vi "Init.vi"(8 "error in (no error)":errorcluster, 11 "Tamer in":refnum<class "Tamer.lvclass">) -> (0 "error out":errorcluster, 3 "Tamer out":refnum<class "Tamer.lvclass">)   [LabVIEW 2020, in "Tamer.lvlib" / "Tamer.lvclass"]
uses:
  Tamer.lvclass
  Tamer Consumer Case Selector.ctl
  Classes/Log/Log.lvclass
  Father of all uServices/Father of all uServices/Father of all uServices.lvclass
  TALOS.lvlib
  Ancestor/Ancestor/Infinite Message Selector.ctl
  Ancestor/Ancestor/Ancestor.lvclass
  C:/Users/marco/Documents/GitHub_Lab/TALOS/talos/Father of all uServices/Father of all uServices/Father of all uServices.lvclass
  C:/Users/marco/Documents/GitHub_Lab/TALOS/talos/Ancestor/Ancestor/Ancestor.lvclass
  C:/Users/marco/Documents/GitHub_Lab/TALOS/builds/Actor Framework PPL/Actor Framework.lvlibp/1abvi3w/vi.lib/ActorFramework/Actor/Actor.lvclass
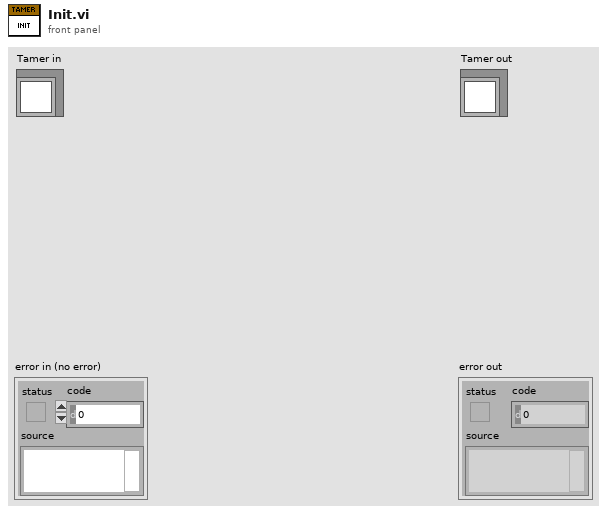
[diagram p1: front panel]
types:
  T1 = typedef "Tamer.lvlib/Tamer.lvclass/Tamer Consumer Case Selector.ctl" = enum16{"New schedule", "Initiate RUN", "Parse Schedules", "Script Checker", "Banana after Quality Check", "Update Crit Lvl", "Propagate Banana", "Reply from Guardian", "Reply from uService", "Timeout of RUN", "uService Replies Check", "Update from Monkey", "Monkey Died", "Reschedule", "Rerun", "Stop DAQ", "Stop Schedule", "Skip Run", "Kill Process", "Update GV"}
  T2 = typedef "TALOS.lvlib/Ancestor.lvlib/Ancestor.lvclass/Infinite Message Selector.ctl" = enum16{"Start", "Stop", "Check", "Flush (Stop all)", "Init"}
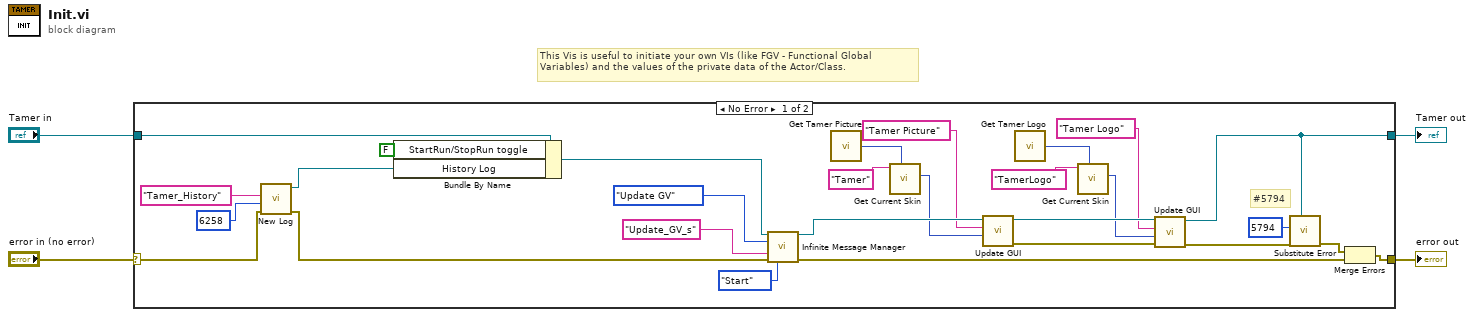
[diagram p0: block diagram]
diagram:
  # "This Vis is useful to initiate your own VIs (like FGV - Functional Global Variables) and the values of the private data of the Actor/Class."
  n1 = case shown="No Error" "error in (no error)" {
    selector: "error in (no error)" -> [w19 w33]
    tunnel: "Tamer in" -> [w24 w34]
    tunnel: [w6 w34] -> w4
    tunnel: [w32 w33] -> w3
    frame No Error {
      # "#5794"
      n2 = call "New Log.vi"("error in (no error)"=w19, "Specific Error Code"=6258, "Name"="Tamer_History") -> ("error out"=w18:errorcluster, "Log out"=w20:refnum<class "Log.lvclass">)  [unwired: 7 in]
      n3 = Bundle By Name(cluster=w24, "StartRun/StopRun toggle"=FALSE ("StartRun already given?"), "History Log"=w20) -> (w25:refnum<class "Tamer.lvclass">)
      n4 = call-dynamic "Infinite Message Manager.vi"("Father of all uServices in"=w25, "Consumer Case Selector"=Tamer_Consumer_Case_Selector."Update GV" ("Monkey Consumer Case Selector"), "Tau parameter"="Update_GV_s", "error in (no error)"=w18, "Infinite Message Selector"=Infinite_Message_Selector."Start") -> ("Father of all uServices out"=w27:refnum<class "Tamer.lvclass">, "error out"=w28:errorcluster)  [unwired: 8 in, 1 out]
      n5 = call "Get Tamer Picture.vi"() -> ("Tamer"=w11:picture)
      n6 = call "Get Current Skin.vi"("default"=w11, "Object"="Tamer") -> ("Picture with skin"=w14:picture)  [unwired: 4 in, 2 out]
      n7 = call "Update GUI.vi"("Data"=w14, "GUI Item Name"="Tamer Picture", "uService Template in"=w27) -> ("error out"=w12:errorcluster, "uService Template out"=w13:refnum<class "Tamer.lvclass">)  [unwired: 7 in]
      n8 = call "Get Tamer Logo.vi"() -> ("Tamer Logo"=w9:picture)
      n9 = call "Get Current Skin.vi"("default"=w9, "Object"="TamerLogo") -> ("Picture with skin"=w8:picture)  [unwired: 4 in, 2 out]
      n10 = call "Update GUI.vi"("error in (no error)"=w12, "Data"=w8, "GUI Item Name"="Tamer Logo", "uService Template in"=w13) -> ("error out"=w5:errorcluster, "uService Template out"=w6:refnum<class "Tamer.lvclass">)  [unwired: 6 in]
      n11 = call "Substitute Error.vi"("LabVIEW Object"=w6, "error in (no error)"=w5, "Error Code"=5794) -> ("error out"=w31:errorcluster)  [unwired: 8 in]
      n12 = Merge Errors(w31, w28) -> (w32:errorcluster)
    }
    frame Error {
    }
  }
  "error out" <- w3
  "Tamer out" <- w4
